vi "ep_Static File Descr Inf to String.vi"(8 "error in":errorcluster, 11 "task in":T1={"file refnums"=[], "Data Object"=refnum, "config info"={"station_name"="", "rec_dev_id"="", "rev_year"=1999.0, "TT"=0, "##A"=0, "##D"=0, "analog channel info"=[], "status channel info"=[], "lf"=-inf, "nrates"=65535, "samp info"=[], "initial timestamp"=timestamp(0 s since 1904-01-01), "trigger timestamp"=timestamp(0 s since 1904-01-01), "ft"=enum."Binary", "timemult"=1.0}, "public inf content"={"Source"="", "Record Type"=enum."Fault", "Phase ID"="", "Event Description"="", "Device ID"="", "Distance of Fault"=-1.0, "Distance Unit"=enum."Miles", "Max_Current"=inf, "Min_Current"=-inf, "Max_Voltage"=inf, "Min_Voltage"=-inf, "EventNoteCount"=0, "Event Information"=[]}, "private inf content"=[], "internal buffers"={"start index"=1, "config to public inf"=enum."disabled", "static config info"="", "static file_des record inf"="", "static file_des channel inf"="", "public inf"="", "private inf"=""}} {"public inf content"."Event Information"."min sample number" max=9999999999; "public inf content"."Event Information"."max sample number" max=9999999999; "config info"."nrates" max=999; "config info"."status channel info"."Dn" min=1 max=999999; "config info"."analog channel info"."An" min=1 max=999999; "config info"."trigger timestamp" format="%<%H:%M:%S%6u\n%d/%m/%Y>T"; "config info"."initial timestamp" format="%<%H:%M:%S%6u\n%d/%m/%Y>T"; "config info"."##D" max=999999; "config info"."##A" max=999999; "config info"."TT" min=1 max=999999; "config info"."rev_year" min=1999.0 max=1999.0}) -> (0 "error out":errorcluster, 3 "task out":T1={"file refnums"=[], "Data Object"=refnum, "config info"={"station_name"="", "rec_dev_id"="", "rev_year"=1999.0, "TT"=0, "##A"=0, "##D"=0, "analog channel info"=[], "status channel info"=[], "lf"=-inf, "nrates"=65535, "samp info"=[], "initial timestamp"=timestamp(0 s since 1904-01-01), "trigger timestamp"=timestamp(0 s since 1904-01-01), "ft"=enum."Binary", "timemult"=1.0}, "public inf content"={"Source"="", "Record Type"=enum."Fault", "Phase ID"="", "Event Description"="", "Device ID"="", "Distance of Fault"=-1.0, "Distance Unit"=enum."Miles", "Max_Current"=inf, "Min_Current"=-inf, "Max_Voltage"=inf, "Min_Voltage"=-inf, "EventNoteCount"=0, "Event Information"=[]}, "private inf content"=[], "internal buffers"={"start index"=1, "config to public inf"=enum."disabled", "static config info"="", "static file_des record inf"="", "static file_des channel inf"="", "public inf"="", "private inf"=""}} {"public inf content"."Event Information"."min sample number" max=9999999999; "public inf content"."Event Information"."max sample number" max=9999999999; "config info"."nrates" max=999; "config info"."status channel info"."Dn" min=1 max=999999; "config info"."analog channel info"."An" min=1 max=999999; "config info"."trigger timestamp" format="%<%H:%M:%S%6u\n%d/%m/%Y>T"; "config info"."initial timestamp" format="%<%H:%M:%S%6u\n%d/%m/%Y>T"; "config info"."##D" max=999999; "config info"."##A" max=999999; "config info"."TT" min=1 max=999999; "config info"."rev_year" min=1999.0 max=1999.0})   [LabVIEW 2014, in "NI_EP_COMTRADE.lvlib"]
uses:
  <vilib>/addons/Electrical Power/File IO/NI_EP_COMTRADE.lvlib
  <vilib>/addons/Electrical Power/File IO/COMTRADE/typedefs/ep_Task.ctl
  <vilib>/addons/Electrical Power/File IO/COMTRADE/typedefs/ep_Config Info.ctl
  <vilib>/addons/Electrical Power/File IO/COMTRADE/typedefs/ep_Analog Channel Info.ctl
  <vilib>/addons/Electrical Power/File IO/COMTRADE/typedefs/ep_Status Channel Info.ctl
  <vilib>/addons/Electrical Power/File IO/COMTRADE/typedefs/ep_File Format.ctl
  <vilib>/addons/Electrical Power/File IO/COMTRADE/typedefs/ep_Public Inf Content.ctl
  <vilib>/addons/Electrical Power/File IO/COMTRADE/typedefs/ep_Public Event Inf.ctl
  <vilib>/addons/Electrical Power/File IO/COMTRADE/typedefs/ep_Private Inf Content.ctl
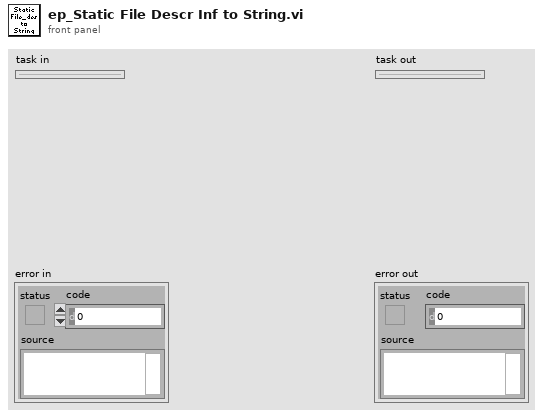
[diagram p1: front panel]
types:
  T1 = typedef "NI_EP_COMTRADE.lvlib/ep_Task.ctl" = cluster{"file refnums":refnum<file>[], "Data Object":refnum<k20>, "config info":T2, "public inf content":T6, "private inf content":T8, "internal buffers":cluster{"start index":u32, "config to public inf":enum16{"disabled", "enabled", "buffered"}, "static config info":string, "static file_des record inf":string, "static file_des channel inf":string, "public inf":string, "private inf":string}}
  T2 = typedef "NI_EP_COMTRADE.lvlib/ep_Config Info.ctl" = cluster{"station_name":string, "rec_dev_id":string, "rev_year":dbl, "TT":u32, "##A":u32, "##D":u32, "analog channel info":T3[], "status channel info":T4[], "lf":sgl, "nrates":u16, "samp info":cluster{"samp":sgl, "endsamp":u32}[], "initial timestamp":timestamp, "trigger timestamp":timestamp, "ft":T5, "timemult":sgl}
  T3 = typedef "NI_EP_COMTRADE.lvlib/ep_Analog Channel Info.ctl" = cluster{"An":u32, "ch_id":string, "ph":string, "ccbm":string, "uu":string, "a":sgl, "b":sgl, "skew":sgl, "min":i32, "max":i32, "primary":sgl, "secondary":sgl, "PS":enum16{"P", "S"}}
  T4 = typedef "NI_EP_COMTRADE.lvlib/ep_Status Channel Info.ctl" = cluster{"Dn":u32, "ch_id":string, "ph":string, "ccbm":string, "Y":bool}
  T5 = typedef "NI_EP_COMTRADE.lvlib/ep_File Format.ctl" = enum16{"ASCII", "Binary"}
  T6 = typedef "NI_EP_COMTRADE.lvlib/ep_Public Inf Content.ctl" = cluster{"Source":string, "Record Type":enum16{"Fault", "Unknown", "Misoperation", "Close", "Trip", "Reclose", "Power swing", "Simulation"}, "Phase ID":string, "Event Description":string, "Device ID":string, "Distance of Fault":dbl, "Distance Unit":enum16{"Miles", "Kilometers", "Percent of line", "Percent of setting", "Ohms"}, "Max_Current":dbl, "Min_Current":dbl, "Max_Voltage":dbl, "Min_Voltage":dbl, "EventNoteCount":u32, "Event Information":T7[]}
  T7 = typedef "NI_EP_COMTRADE.lvlib/ep_Public Event Inf.ctl" = cluster{"channel number":u32, "max value":dbl, "min value":dbl, "max sample number":u64, "min sample number":u64, "max sample text":string[], "min sample text":string[]}
  T8 = typedef "NI_EP_COMTRADE.lvlib/ep_Private Inf Content.ctl" = cluster{"Section Header":string, "Entry Names":string[], "Entry Values":string[]}[]
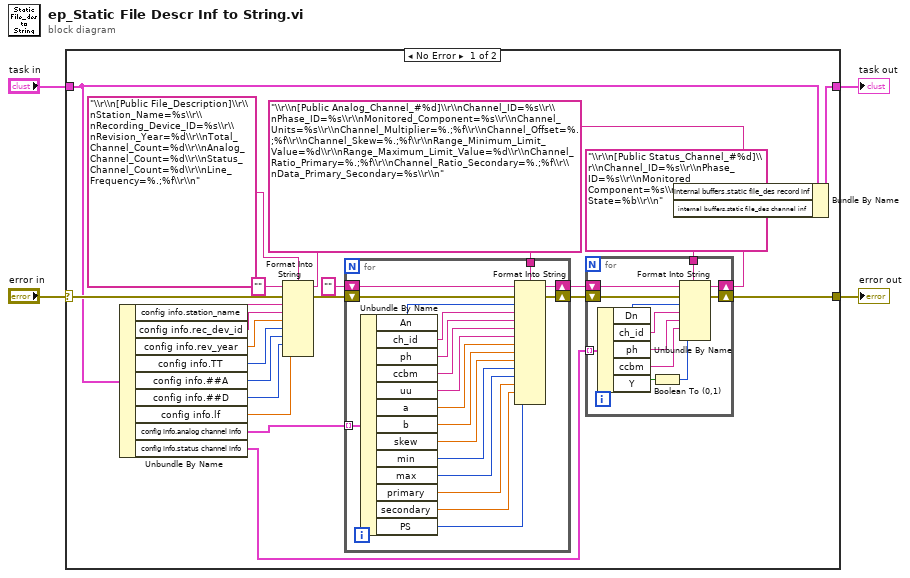
[diagram p0: block diagram]
diagram:
  n1 = case shown="No Error" "error in" {
    selector: "error in" -> [w18 w60]
    tunnel: "task in" -> [w15 w59]
    tunnel: [w16 w60] -> w1
    tunnel: [w14 w59] -> w3
    frame No Error {
      n2 = Unbundle By Name(w15) -> ("config info.station_name"=w19:string, "config info.rec_dev_id"=w24:string, "config info.rev_year"=w5:dbl, "config info.TT"=w20:u32, "config info.##A"=w21:u32, "config info.##D"=w9:u32, "config info.lf"=w8:sgl, "config info.analog channel info"=w10:T3[], "config info.status channel info"=w23:T4[])
      n3 = Format Into String(format string="\\r\\n[Public File_Description]\\r\\nStation_Name=%s\\r\\nRecording_Device_ID=%s\\r\\nRevision_Year=%d\\r\\nTotal_Channel_Count=%d\\r\\nAnalog_Channel_Count=%d\\r\\nStatus_Channel_Count=%d\\r\\nLine_Frequency=%.;%f\\r\\n", initial string="", error in=w18, w19, w24, w5, w20, w21, w9, w8) -> (resulting string=w11:string, error out=w22:errorcluster)
      n4 = for {
        tunnel: w10 -> [w58] mode=indexing
        shift-right: [w56] -> w26
        shift-left: "" -> [w57]
        shift-right: [w54] -> w25
        shift-left: w22 -> [w55]
        tunnel: "\\r\\n[Public Analog_Channel_#%d]\\r\\nChannel_ID=%s\\r\\nPhase_ID=%s\\r\\nMonitored_Component=%s\\r\\nChannel_Units=%s\\r\\nChannel_Multiplier=%.;%f\\r\\nChannel_Offset=%.;%f\\r\\nChannel_Skew=%.;%f\\r\\nRange_Minimum_Limit_Value=%d\\r\\nRange_Maximum_Limit_Value=%d\\r\\nChannel_Ratio_Primary=%.;%f\\r\\nChannel_Ratio_Secondary=%.;%f\\r\\nData_Primary_Secondary=%s\\r\\n" ("format string") -> [w40]
        n5 = Unbundle By Name(w58) -> ("An"=w52:u32, "ch_id"=w53:string, "ph"=w48:string, "ccbm"=w49:string, "uu"=w46:string, "a"=w45:sgl, "b"=w44:sgl, "skew"=w47:sgl, "min"=w42:i32, "max"=w43:i32, "primary"=w41:sgl, "secondary"=w51:sgl, "PS"=w50:enum16{"P", "S"})
        n6 = Format Into String(format string=w40, initial string=w57, error in=w55, w52, w53, w48, w49, w46, w45, w44, w47, w42, w43, w41, w51, w50) -> (resulting string=w56:string, error out=w54:errorcluster)
      }
      n7 = for {
        tunnel: w23 -> [w39] mode=indexing
        shift-right: [w33] -> w13
        shift-left: w26 -> [w34]
        shift-right: [w29] -> w16
        shift-left: w25 -> [w30]
        tunnel: "\\r\\n[Public Status_Channel_#%d]\\r\\nChannel_ID=%s\\r\\nPhase_ID=%s\\r\\nMonitored_Component=%s\\r\\nNormal_State=%b\\r\\n" ("format string") -> [w28]
        n8 = Unbundle By Name(w39) -> ("Dn"=w38:u32, "ch_id"=w37:string, "ph"=w36:string, "ccbm"=w35:string, "Y"=w32:bool)
        n9 = Boolean To (0,1)(Boolean=w32) -> (0, 1=w31:i16)
        n10 = Format Into String(format string=w28, initial string=w34, error in=w30, w38, w37, w36, w35, w31) -> (resulting string=w33:string, error out=w29:errorcluster)
      }
      n11 = Bundle By Name(cluster=w15, "internal buffers.static file_des record inf"=w11, "internal buffers.static file_des channel inf"=w13) -> (w14:T1)
    }
    frame Error {
    }
  }
  "task out" <- w3
  "error out" <- w1
